vi "Save Load Mass Storage Waveform.vi"(6 "Edit Memory (0: Edit Memory)":i32(ring) items=["Edit Memory", "Edit Memory 1", "Edit Memory 2"], 8 "error in (no error)":errorcluster, 9 "File Name (TEK001.TFW)":string="TEK001.TFW", 10 "Operation Select (0: Load Waveform)":i32(ring) items=["Load Waveform", "Store Waveform"], 11 "VISA resource name":refnum<visa-resource-name>) -> (0 "error out":errorcluster, 3 "VISA resource name out":refnum<visa-resource-name>)   [LabVIEW 2013, in "Tektronix AFG 3000 Series.lvlib"]
doc: "Saves or loads an Edit Memory waveform data to mass storage file. \n\n<B>Note:</B>\n \n(1) This VI is only applicable for AFG 3KC series.\n(2) If the file format is different, this VI causes an error."
uses:
  Tektronix AFG 3000 Series.lvlib
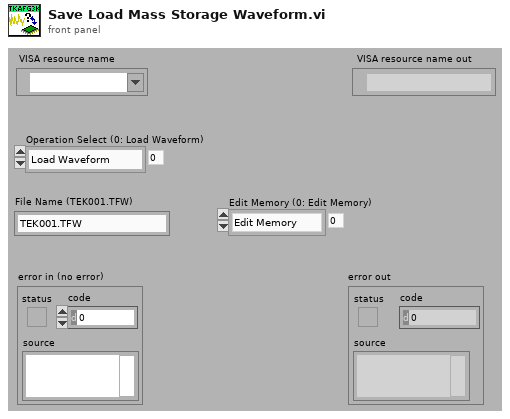
[diagram p1: front panel]
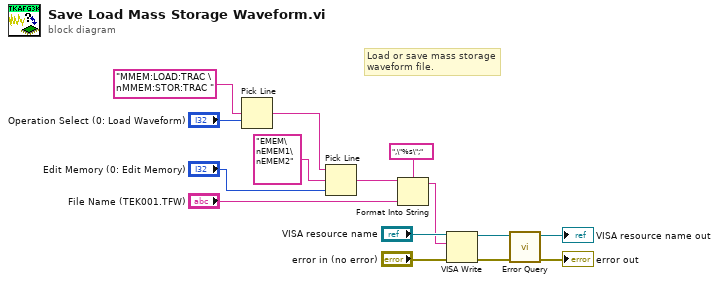
[diagram p0: block diagram]
diagram:
  # "Load or save mass storage \nwaveform file."
  n1 = Pick Line(multi-line string="MMEM:LOAD:TRAC \nMMEM:STOR:TRAC " ("string (\"\")"), line index="Operation Select (0: Load Waveform)") -> (output string=w2:string)  [unwired: 1 in]
  n2 = Pick Line(string ("")=w2, multi-line string="EMEM\nEMEM1\nEMEM2" ("string (\"\")"), line index="Edit Memory (0: Edit Memory)") -> (output string=w3:string)
  n3 = Format Into String(format string=",\"%s\";" ("string (\"\")"), initial string=w3, "File Name (TEK001.TFW)") -> (resulting string=w6:string)  [unwired: 1 in, 1 out]
  n4 = VISA Write(VISA resource name="VISA resource name", write buffer=w6, error in (no error)="error in (no error)") -> (VISA resource name out=w15:refnum<visa-resource-name>, error out=w14:errorcluster)  [unwired: 1 out]
  n5 = call "Error Query.vi"("error in (no error)"=w14, "VISA resource name"=w15) -> ("error out"=→"error out":errorcluster, "VISA resource name out"=→"VISA resource name out":refnum<visa-resource-name>)  [unwired: 6 in, 2 out]
